vi "Detecction_warning_anterior (SubVI).vi"(10 "warnings table in":T1(array[cluster]), 11 "Index in":i32) -> (2 "Index Out":i32, 3 "Add W?":bool)   [LabVIEW 2022 SP3]
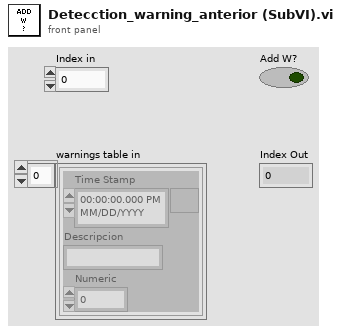
[diagram p1: front panel]
types:
  T1 = cluster{"Time Stamp":timestamp, "Descripcion":string, "Numeric":i32}[]
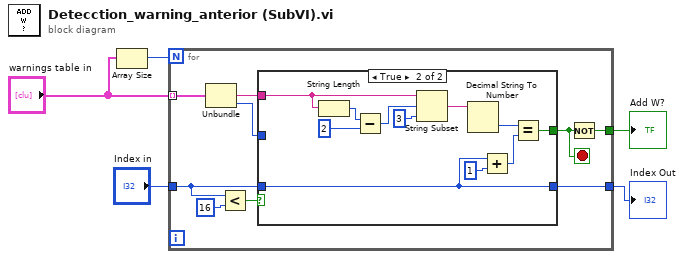
[diagram p0: block diagram]
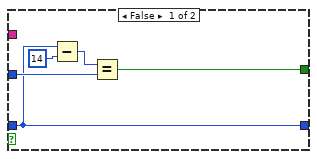
[diagram p2: hidden frame]
diagram:
  n1 = Array Size(array="warnings table in") -> (size(s)=w5:i32)
  n2 = for {
    N: w5 -> [_]
    tunnel: "warnings table in" -> [w11] mode=indexing
    tunnel: "Index in" -> [w9]
    tunnel: [w6] -> w2
    tunnel: [w14] -> w1
    stop <- w8 stop-if-true
    n3 = Unbundle(w11) -> ("Descripcion"=w7:string, "Numeric"=w10:i32)  [unwired: 1 out]
    n4 = Less?(x=w9, y=16) -> (x < y?=w12:bool)
    n5 = case shown="True" w12 {
      tunnel: w10 -> [w19 _]
      tunnel: w9 -> [w16 w27]
      tunnel: [w18 w28] -> w8
      tunnel: w7 -> [_ w20]
      tunnel: [w16 w27] -> w6
      frame False {
        n6 = Subtract(x=w16, y=14) -> (x-y=w17:i32)
        n7 = Equal?(x=w17, y=w19) -> (x = y?=w18:bool)
      }
      frame True {
        n8 = String Length(string=w20) -> (length=w24:i32)
        n9 = Subtract(x=w24, y=2) -> (x-y=w25:i32)
        n10 = String Subset(string=w20, offset (0)=w25, length (rest)=3 ("length (rest)")) -> (substring=w21:string)
        n11 = Decimal String To Number(string=w21) -> (number=w26:i32)  [unwired: 2 in, 1 out]
        n12 = Add(x=w27, y=1) -> (x+y=w29:i32)
        n13 = Equal?(x=w26, y=w29) -> (x = y?=w28:bool)
      }
    }
    n14 = Not(x=w8) -> (.not. x?=w14:bool)
  }
  "Add W?" <- w1
  "Index Out" <- w2
